vi "EX_TEST.vi"() -> ()   [LabVIEW 2017]
panel:
  out "读取缓冲区":string
  in  "停止":bool
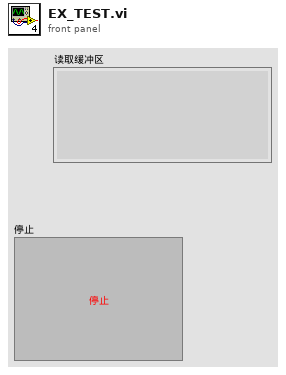
[diagram p1: front panel]
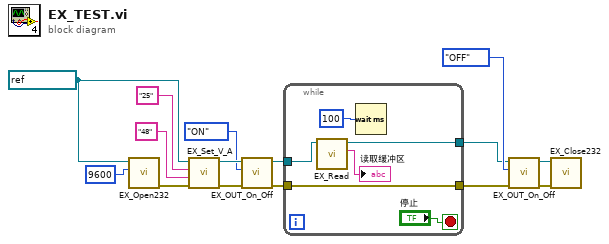
[diagram p0: block diagram]
diagram:
  w12 = refnum<visa-resource-name> "COM12" ("VISA resource name")
  n1 = call "EX_Open232.vi"("baud rate (9600)"=u32 9600, "VISA resource name"=w12) -> ("error out"=w10:errorcluster)  [unwired: 8 in, 1 out]
  n2 = call "EX_Set_V_A.vi"("错误输入（无错误）"=w10, "current"="48", "voltage"="25", "VISA resource name"=w12) -> ("error out"=w9:errorcluster, "VISA资源名称输出"=w11:refnum<visa-resource-name>)  [unwired: 6 in]
  n3 = call "EX_OUT_On_Off.vi"("错误输入（无错误）"=w9, "Mode"=enum16{"ON", "OFF"}."ON", "VISA resource name"=w11) -> ("error out"=w8:errorcluster, "VISA资源名称输出"=w2:refnum<visa-resource-name>)  [unwired: 7 in]
  n4 = while {
    tunnel: w8 -> [w19]
    tunnel: [w19] -> w6
    tunnel: w2 -> [w18]
    tunnel: [w17] -> w1
    stop <- "停止" stop-if-true
    n5 = call "EX_Read.vi"("VISA resource name"=w18) -> ("读取缓冲区"=→"读取缓冲区":string, "VISA资源名称输出"=w17:refnum<visa-resource-name>)  [unwired: 8 in, 1 out]
    n6 = Wait (ms)(milliseconds to wait=u32 100 ("等待时间（毫秒）")) -> ()  [unwired: 1 out]
  }
  n7 = call "EX_OUT_On_Off.vi"("错误输入（无错误）"=w6, "Mode"=enum16{"ON", "OFF"}."OFF", "VISA resource name"=w1) -> ("error out"=w5:errorcluster, "VISA资源名称输出"=w4:refnum<visa-resource-name>)  [unwired: 7 in]
  n8 = call "EX_Close232.vi"("error in (no error)"=w5, "VISA resource name"=w4) -> ()  [unwired: 9 in, 1 out]
